vi "ReadConfig.vi"(8 "error in (no error)":errorcluster, 11 "PmuBase in":refnum<class "PmuBase.lvclass">) -> (0 "error out":errorcluster, 2 "Config":variant, 3 "PmuBase out":refnum<class "PmuBase.lvclass">)   [LabVIEW 2014, in "SensorPlugins.lvlib" / "PmuBase.lvclass"]
uses:
  PmuBase.lvclass
  PmuBase.lvclass/PmuBase.ctl
  Accessors/Read PmuConfig.vi
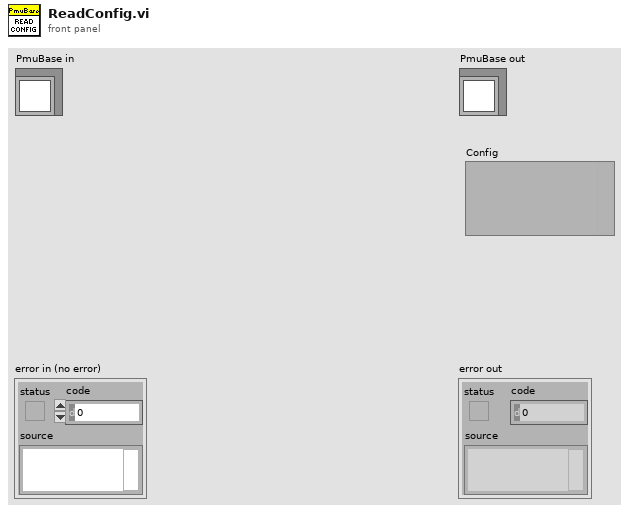
[diagram p1: front panel]
types:
  T1 = typedef "SensorPlugins.lvlib/PmuBase.lvclass/PmuConfig.ctl" = cluster{"Class":enum16{"M", "P"}, "Fs":i32, "F0":i32, "FSamp":i32, "SettlingTime":dbl, "T0":ext}
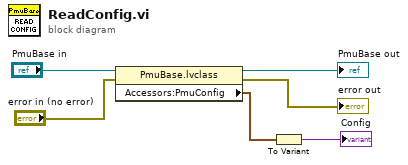
[diagram p0: block diagram]
diagram:
  n1 = property class="PmuBase.lvclass"(reference="PmuBase in", error in="error in (no error)") -> (reference out=→"PmuBase out":refnum<class "PmuBase.lvclass">, error out=→"error out":errorcluster, "Accessors:PmuConfig"=w3:T1)
  n2 = To Variant(anything=w3) -> (Variant=→"Config":variant)
